vi "[Global].vi"() -> ()   [LabVIEW 2023, in "Plugin Generator.lvlib"]
uses:
  Plugin Generator.lvlib
panel:
  out "Time Stamp":timestamp
  out "Progress":string
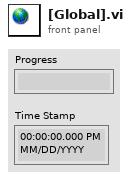
[diagram p1: front panel]
diagram:
